vi "Is Display Active.vi"(8 "error in (no error)":errorcluster, 10 "create if not found? (T)":bool) -> (0 "error out":errorcluster, 2 "Display Active":bool, 3 "Display Active Queue":refnum<queue>)   [LabVIEW 2018, in "Assert API Components.lvlib" / "Assert Display.lvlib"]
uses:
  Assert Display.lvlib
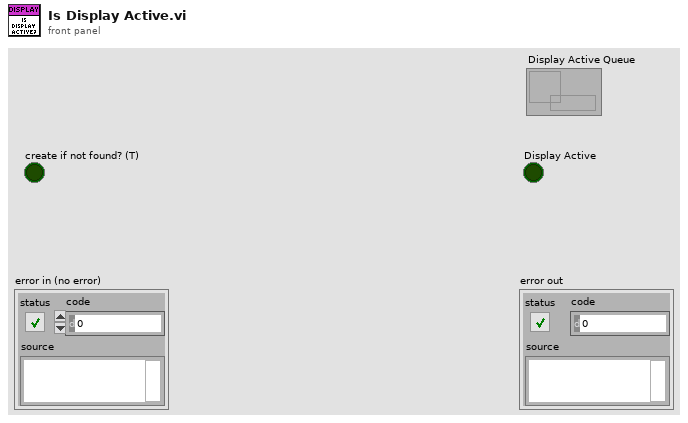
[diagram p1: front panel]
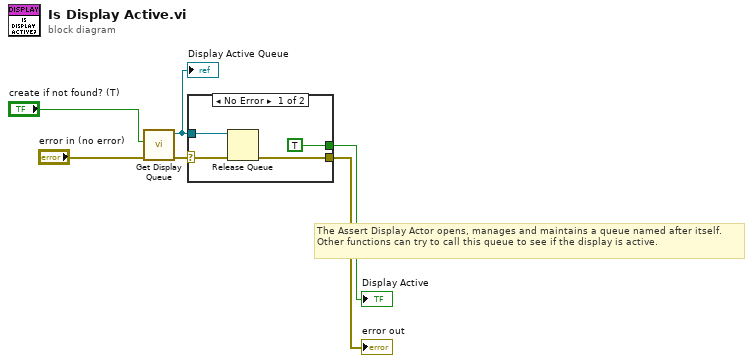
[diagram p0: block diagram]
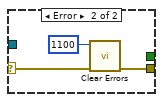
[diagram p2: hidden frame]
diagram:
  # "The Assert Display Actor opens, manages and maintains a queue named after itself. Other functions can try to call this queue to see if the display is active."
  n1 = call "Get Display Queue.vi"("error in (no error)"="error in (no error)", "create if not found? (T)"="create if not found? (T)") -> ("error out"=w5:errorcluster, "Queue out"=w4:refnum<queue>)  [unwired: 8 in]
  "Display Active Queue" <- w4
  n2 = case shown="No Error" w5 {
    selector: w5 -> [w10 w12]
    tunnel: w4 -> [w9 _]
    tunnel: [w8 w11] -> w3
    tunnel: [TRUE _] -> w2
    frame No Error {
      n3 = Release Queue(queue=w9, error in (no error)=w10) -> (error out=w8:errorcluster)  [unwired: 1 in, 2 out]
    }
    frame Error {
      n4 = call <vilib>:"Clear Errors.vi"("error in (no error)"=w12, "specific error code to clear (0: all)"=1100) -> ("error out"=w11:errorcluster)  [unwired: 4 in, 1 out]
    }
  }
  "error out" <- w3
  "Display Active" <- w2
